vi "to string.vi"(8 "error in":errorcluster, 11 "Daqmx Module configuration in":refnum<class "Daqmx Module configuration.lvclass">) -> (0 "error out":errorcluster, 1 "data":string, 2 "version":string, 3 "Daqmx Module configuration out":refnum<class "Daqmx Module configuration.lvclass">)   [LabVIEW 2014, in "DAQmx Module Configuration.lvclass"]
doc: "Provides an interface for saving a module configuration to a file or other serialized data source. It is recommended that all children of this class store data in two sets--data required for its own initialization, and any data required for parent initialization--and that each implementation uses the <b>Call Parent Method</b> primitive to serialize parent information."
uses:
  Daqmx Module configuration.lvclass
  Daqmx Module configuration.lvclass/Daqmx Module configuration.ctl
  current version.vi
  <vilib>/NI/Tag Bus Module Framework/module configuration/TBM module configuration.lvclass
  <vilib>/NI/Tag Bus Module Framework/channel/TBM channel.lvclass
  <vilib>/NI/Configuration Framework/serializable configuration/NISE_CEF_serializable configuration.lvclass
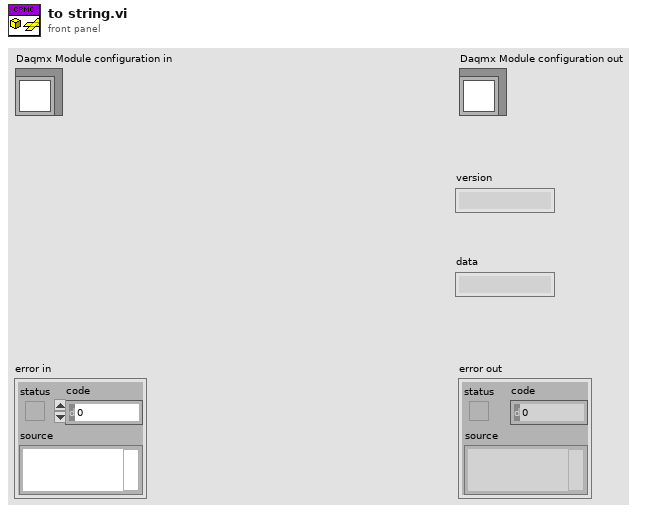
[diagram p1: front panel]
types:
  T1 = typedef "DAQmx Module Configuration1.lvclass/Line.ctl" = cluster{"channel":refnum<class "TBM channel.lvclass">, "Physical Channel":string, "Measurement Type":T2, "Parameters":T3}
  T2 = typedef "DAQmx Module Configuration1.lvclass/Measurement Type.ctl" = enum16{"Digital Input", "Digital Output", "Voltage Input", "Voltage Output", "Current Input", "Current Output", "RTD", "Thermocouple", "Strain"}
  T3 = typedef "DAQmx Module Configuration1.lvclass/Parameters.ctl" = cluster{"Digital Config":cluster{"Invert Lines?":bool}, "Voltage Config":cluster{"Maximum Value (V)":dbl, "Minimum Value (V)":dbl, "in terminal configuration (V)":i32, "out terminal configuration (V)":i32}, "Current Config":cluster{"Maximum Value (A)":dbl, "Minimum Value (A)":dbl, "shunt resistor location":i32, "input terminal configuration (C)":i32, "external shunt resistor value":dbl}, "RTD Config":cluster{"Maximum Value (°C)":dbl, "Minimum Value (°C)":dbl, "resistance configuration":i32, "r0":dbl, "current excitation value":dbl, "rtd type":i32, "current excitation source":i32}, "Thermocouple Config":cluster{"Minimum Value (C)":dbl, "Maximum Value (C)":dbl, "thermocouple type":i32, "cjc source":i32, "cjc value":dbl}, "Strain Config":cluster{"Maximum Value":dbl, "Minimum Value":dbl, "bridge information":cluster{"strain configuration":i32, "lead wire resistance":dbl, "initial bridge voltage":dbl, "voltage excitation source":i32, "voltage excitation value":dbl}, "strain gage information":cluster{"gage factor":dbl, "nominal gage resistance":dbl, "poisson ratio":dbl}}}
  T4 = cluster{"strain configuration":i32, "lead wire resistance":dbl, "initial bridge voltage":dbl, "voltage excitation source":i32, "voltage excitation value":dbl}
  T5 = cluster{"gage factor":dbl, "nominal gage resistance":dbl, "poisson ratio":dbl}
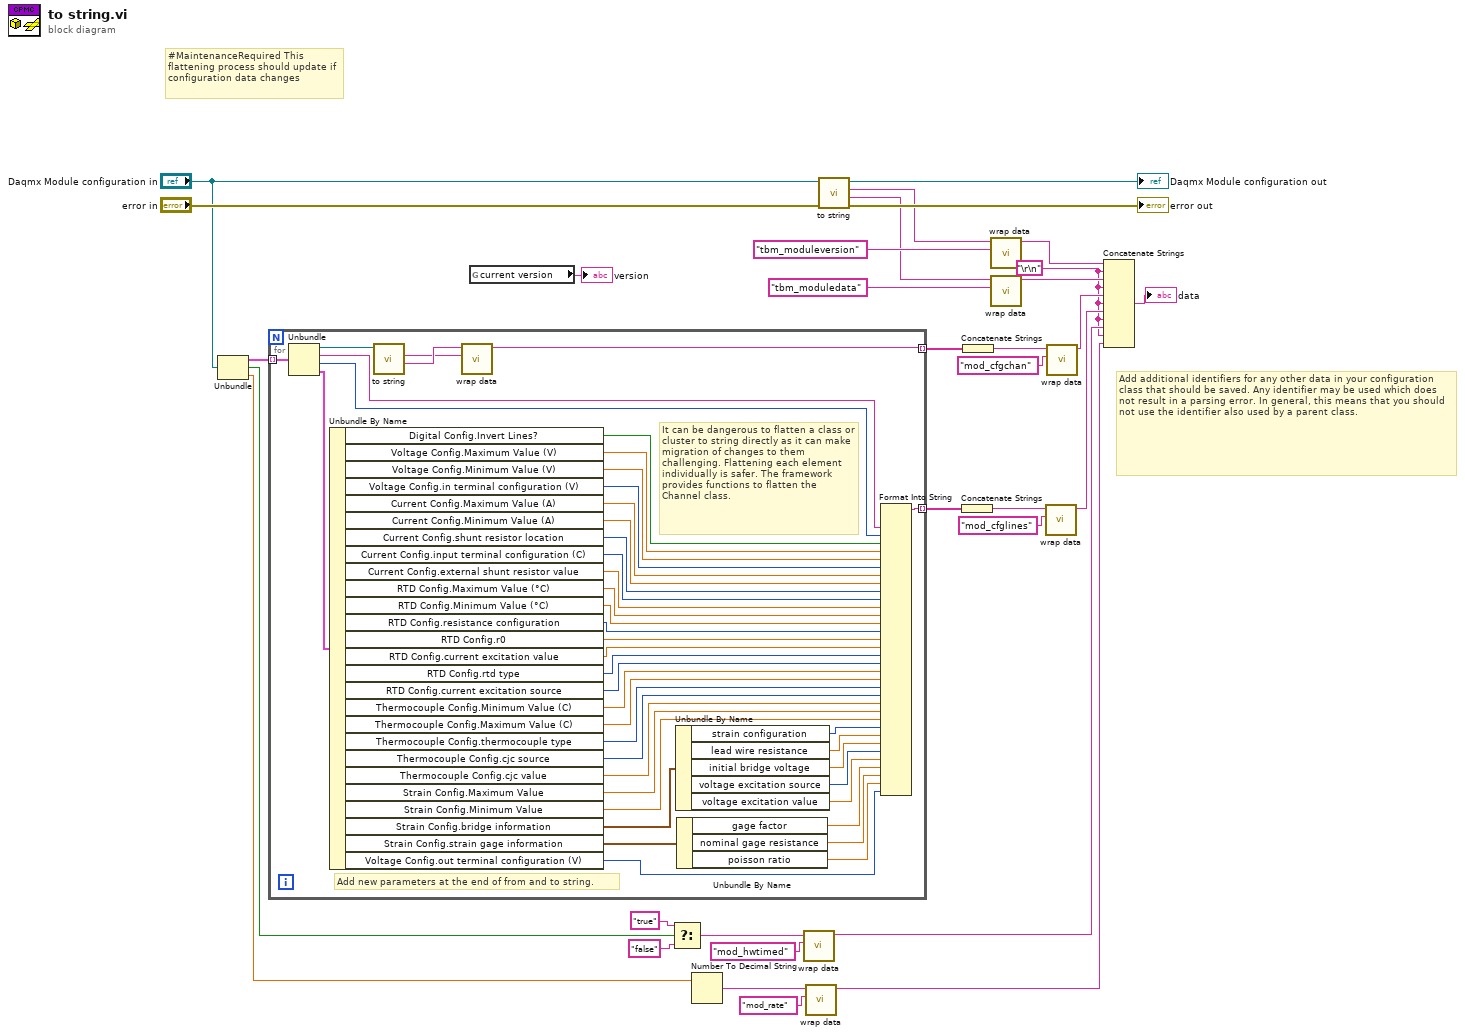
[diagram p0: block diagram]
diagram:
  w1 = "\r\n"
  # "Add additional identifiers for any other data in your configuration class that should be saved. Any identifier may be used which does not result in a parsing error. In general, this means that you should not use the identifier also used by a parent class."
  # "#MaintenanceRequired This flattening process should update if configuration data changes"
  n1 = Unbundle("Daqmx Module configuration in") -> (w19:T1[], w6:bool, w2:dbl)
  n2 = for {
    tunnel: w19 -> [w75] mode=indexing
    tunnel: [w72] -> w18 mode=indexing
    tunnel: [w38] -> w13 mode=indexing
    # "Add new parameters at the end of from and to string."
    # "It can be dangerous to flatten a class or cluster to string directly as it can make migration of changes to them challenging. Flattening each element individually is safer. The framework provides functions to flatten the Channel class."
    n3 = Unbundle(w75) -> ("channel"=w74:refnum<class "TBM channel.lvclass">, "Physical Channel"=w36:string, "Measurement Type"=w37:T2, "Parameters"=w39:T3)
    n4 = Unbundle By Name(w39) -> ("Digital Config.Invert Lines?"=w70:bool, "Voltage Config.Maximum Value (V)"=w69:dbl, "Voltage Config.Minimum Value (V)"=w68:dbl, "Voltage Config.in terminal configuration (V)"=w67:i32, "Current Config.Maximum Value (A)"=w66:dbl, "Current Config.Minimum Value (A)"=w65:dbl, "Current Config.shunt resistor location"=w64:i32, "Current Config.input terminal configuration (C)"=w63:i32, "Current Config.external shunt resistor value"=w62:dbl, "RTD Config.Maximum Value (°C)"=w61:dbl, "RTD Config.Minimum Value (°C)"=w60:dbl, "RTD Config.resistance configuration"=w59:i32, "RTD Config.r0"=w58:dbl, "RTD Config.current excitation value"=w57:dbl, "RTD Config.rtd type"=w56:i32, "RTD Config.current excitation source"=w55:i32, "Thermocouple Config.Minimum Value (C)"=w54:dbl, "Thermocouple Config.Maximum Value (C)"=w53:dbl, "Thermocouple Config.thermocouple type"=w52:i32, "Thermocouple Config.cjc source"=w51:i32, "Thermocouple Config.cjc value"=w50:dbl, "Strain Config.Maximum Value"=w49:dbl, "Strain Config.Minimum Value"=w48:dbl, "Strain Config.bridge information"=w35:T4, "Strain Config.strain gage information"=w34:T5, "Voltage Config.out terminal configuration (V)"=w33:i32)
    n5 = call-dynamic "to string.vi"("channel in"=w74) -> ("channel data"=w73:string, "identifier"=w71:string)  [unwired: 7 in, 2 out]
    n6 = call <vilib>:"wrap data.vi"("identifier"=w71, "data to wrap"=w73) -> ("wrapped data"=w72:string)  [unwired: 9 in]
    n7 = Unbundle By Name(w35) -> ("strain configuration"=w47:i32, "lead wire resistance"=w46:dbl, "initial bridge voltage"=w45:dbl, "voltage excitation source"=w44:i32, "voltage excitation value"=w43:dbl)
    n8 = Unbundle By Name(w34) -> ("gage factor"=w42:dbl, "nominal gage resistance"=w41:dbl, "poisson ratio"=w40:dbl)
    n9 = Format Into String(w36, w37, w70, w69, w68, w67, w66, w65, w64, w63, w62, w61, w60, w59, w58, w57, w56, w55, w54, w53, w52, w51, w50, w49, w48, w47, w46, w45, w44, w43, w42, w41, w40, w33) -> (resulting string=w38:string)  [unwired: 3 in, 1 out]
  }
  n10 = global read "current version.vi" "current version"() -> (→"version":string)
  n11 = Select(t="true" ("identifier"), s=w6, f="false" ("identifier")) -> (s? t:f=w7:string)
  n12 = Number To Decimal String(number=w2) -> (decimal integer string=w3:string)  [unwired: 1 in]
  n13 = call <vilib>:"wrap data.vi"("identifier"="mod_hwtimed", "data to wrap"=w7) -> ("wrapped data"=w10:string)  [unwired: 9 in]
  n14 = call <vilib>:"wrap data.vi"("identifier"="mod_rate", "data to wrap"=w3) -> ("wrapped data"=w8:string)  [unwired: 9 in]
  n15 = call-parent "to string.vi"("error in"="error in", "module configuration in"="Daqmx Module configuration in") -> ("error out"=→"error out":errorcluster, "data"=w23:string, "version"=w24:string, "module configuration out"=→"Daqmx Module configuration out":refnum<class "Daqmx Module configuration.lvclass">)  [unwired: 6 in]
  n16 = Concatenate Strings(w13) -> (w15:string)
  n17 = Concatenate Strings(w18) -> (w17:string)
  n18 = call <vilib>:"wrap data.vi"("identifier"="tbm_moduleversion" ("additional identifier"), "data to wrap"=w24) -> ("wrapped data"=w26:string)  [unwired: 9 in]
  n19 = call <vilib>:"wrap data.vi"("identifier"="tbm_moduledata" ("additional identifier"), "data to wrap"=w23) -> ("wrapped data"=w25:string)  [unwired: 9 in]
  n20 = call <vilib>:"wrap data.vi"("identifier"="mod_cfglines", "data to wrap"=w15) -> ("wrapped data"=w12:string)  [unwired: 9 in]
  n21 = call <vilib>:"wrap data.vi"("identifier"="mod_cfgchan", "data to wrap"=w17) -> ("wrapped data"=w20:string)  [unwired: 9 in]
  n22 = Concatenate Strings(w26, w1, w25, w1, w20, w1, w12, w1, w10, w1, w8) -> (→"data":string)
